vi "Main.vi"() -> ()   [LabVIEW 2024]
panel:
  in  "Use Browse for Path Method":bool
  in  "logging folder path 2":path=path "C:/Users/sujain/Desktop/LabVIEW demo/path2"
  in  "logging path 1":path=path "C:/Users/sujain/Desktop/LabVIEW demo/path1"
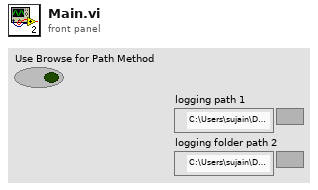
[diagram p1: front panel]
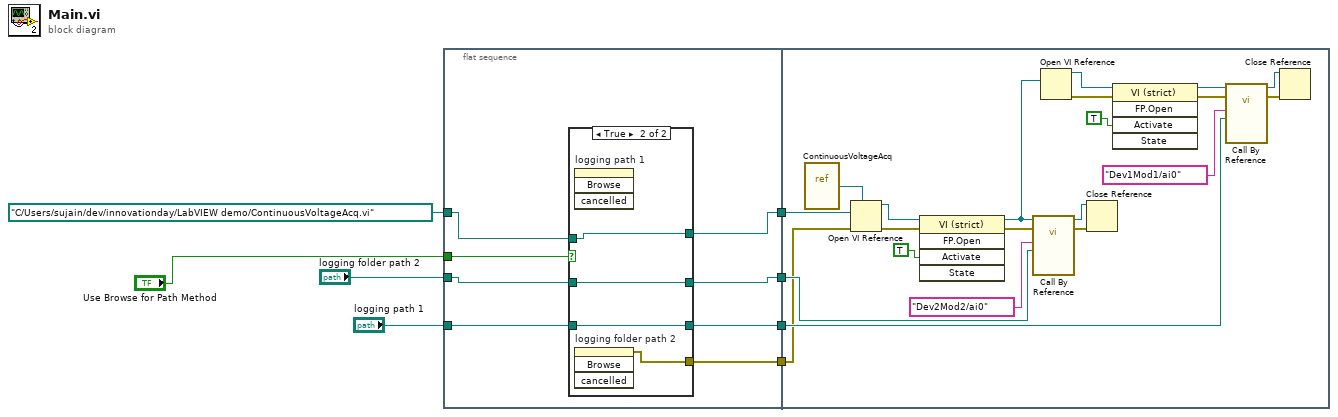
[diagram p0: block diagram]
diagram:
  n1 = flat-sequence {
    tunnel: [w12] -> w8
    tunnel: "logging folder path 2" -> [w15]
    tunnel: [w11] -> w6
    tunnel: "logging path 1" -> [w14]
    tunnel: path "C:/Users/sujain/dev/innovationday/LabVIEW demo/ContinuousVoltageAcq.vi" ("task VI path") -> [w16]
    tunnel: [w13] -> w3
    tunnel: [w10] -> w2
    tunnel: "Use Browse for Path Method" -> [w9]
    tunnel: w8 -> [w31]
    tunnel: w6 -> [w33]
    tunnel: w3 -> [w43]
    tunnel: w2 -> [w24]
    frame #0 {
      n2 = case shown="True" w9 {
        tunnel: w16 -> [w19 w23]
        tunnel: [w19 w23] -> w13
        tunnel: w15 -> [w18 w22]
        tunnel: [w18 w22] -> w12
        tunnel: w14 -> [w17 w21]
        tunnel: [w17 w21] -> w11
        tunnel: [_ w20] -> w10
        frame False {
        }
        frame True {
          n3 = invoke on="logging path 1" class="Path" method="Browse"() -> ()  [unwired: 4 in, 4 out]
          n4 = invoke on="logging folder path 2" class="Path" method="Browse"() -> (error out=w20:errorcluster)  [unwired: 4 in, 3 out]
        }
      }
    }
    frame #1 {
      n5 = vi-ref "ContinuousVoltageAcq.vi"() -> (w44:refnum<vi>)
      n6 = Open VI Reference(type specifier VI Refnum (for type only)=w44, vi path=w43, error in (no error)=w24) -> (vi reference=w41:refnum<vi>, error out=w38:errorcluster)  [unwired: 3 in]
      n7 = invoke class="VI (strict)" method="FP.Open"(reference=w41, error in=w38, "Activate"=TRUE ("Activate?")) -> (reference out=w25:refnum<vi>, error out=w30:errorcluster)  [unwired: 2 in, 3 out]
      n8 = call-by-ref "?"(reference=w25, error in=w30, "logbook folder path"=w31, "Physical Channel"=tag "Dev2Mod2/ai0") -> (reference out=w27:refnum<vi>, error out=w26:errorcluster)  [unwired: 10 in]
      n9 = Open VI Reference(vi path=w25) -> (vi reference=w42:refnum<vi>, error out=w40:errorcluster)  [unwired: 5 in]
      n10 = Close Reference(reference=w27, error in (no error)=w26) -> ()  [unwired: 1 out]
      n11 = invoke class="VI (strict)" method="FP.Open"(reference=w42, error in=w40, "Activate"=TRUE ("Activate?")) -> (reference out=w36:refnum<vi>, error out=w35:errorcluster)  [unwired: 2 in, 3 out]
      n12 = call-by-ref "?"(reference=w36, error in=w35, "logbook folder path"=w33, "Physical Channel"=tag "Dev1Mod1/ai0") -> (reference out=w28:refnum<vi>, error out=w29:errorcluster)  [unwired: 10 in]
      n13 = Close Reference(reference=w28, error in (no error)=w29) -> ()  [unwired: 1 out]
    }
  }
